vi "Assign UUID.vi"(8 "error in (no error)":errorcluster, 11 "Actor Nest in":refnum<class "Actor Nest.lvclass">) -> (0 "error out":errorcluster, 2 "String UUID":string, 3 "Actor Nest out":refnum<class "Actor Nest.lvclass">)   [LabVIEW 2018, in "Actor Nest.lvlib" / "Actor Nest.lvclass"]
uses:
  Actor Nest.lvclass
  Actor Nest.lvclass/Actor Nest.ctl
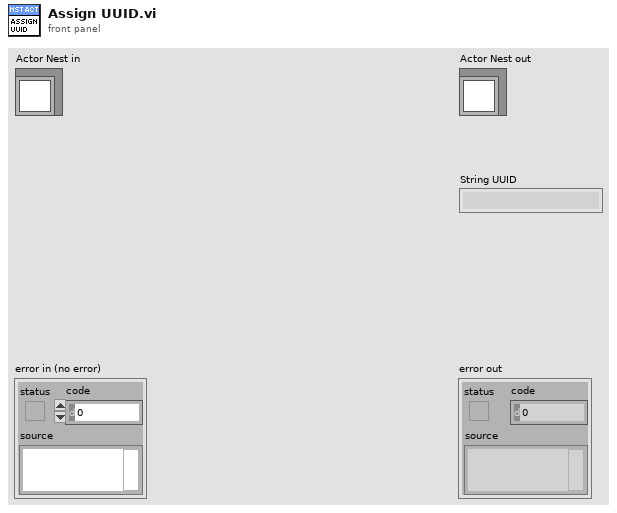
[diagram p1: front panel]
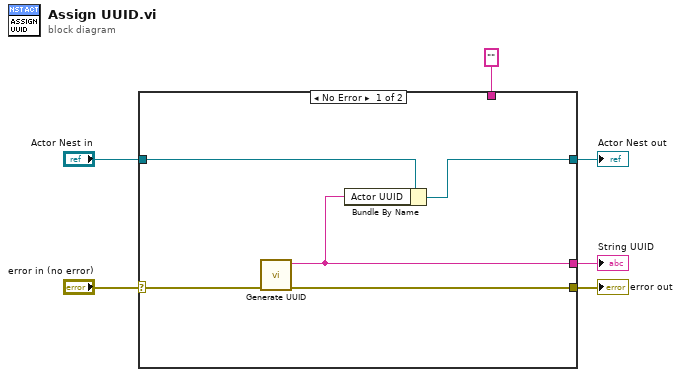
[diagram p0: block diagram]
diagram:
  n1 = case shown="No Error" "error in (no error)" {
    selector: "error in (no error)" -> [w11 w14]
    tunnel: [w8 w14] -> w5
    tunnel: [w9 w13] -> w3
    tunnel: "Actor Nest in" -> [w10 w13]
    tunnel: [w7 w12] -> w2
    tunnel: "" ("String UUID") -> [_ w12]
    frame No Error {
      n2 = call "Generate UUID.vi"("error in (no error)"=w11) -> ("error out"=w8:errorcluster, "String UUID"=w7:string)  [unwired: 8 in, 1 out]
      n3 = Bundle By Name(cluster=w10, "Actor UUID"=w7) -> (w9:refnum<class "Actor Nest.lvclass">)
    }
    frame Error {
    }
  }
  "error out" <- w5
  "Actor Nest out" <- w3
  "String UUID" <- w2
